vi "Remove Empty Strings.vi"(0 "Instrument Types Out in":string[](array[string])) -> (4 "Instrument Types Out out":string[](array[string]))   [LabVIEW 2021, in "Migrator.lvlib"]
uses:
  Migrator.lvlib
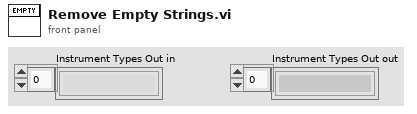
[diagram p1: front panel]
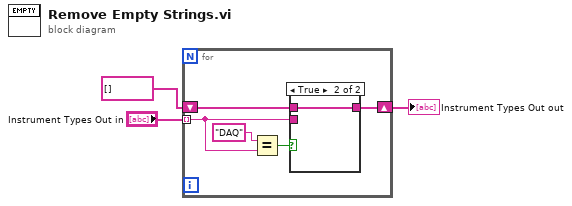
[diagram p0: block diagram]
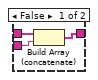
[diagram p2: hidden frame]
diagram:
  n1 = for {
    tunnel: "Instrument Types Out in" -> [w4] mode=indexing
    shift-right: [w6] -> w3
    shift-left: string[] [] -> [w5]
    n2 = Equal?(x="DAQ", y=w4) -> (x = y?=w7:bool)
    n3 = case shown="True" w7 {
      tunnel: [w10 w12] -> w6
      tunnel: w5 -> [w9 w12]
      tunnel: w4 -> [w11 _]
      frame False {
        n4 = Build Array (concatenate)(w9, w11) -> (w10:string[])
      }
      frame True {
      }
    }
  }
  "Instrument Types Out out" <- w3
